vi "Compare_One_Term_Heirarchy.vi"   [LabVIEW 2021]
uses:
  Support/Equal 0/DBL/Equal 0_DBL.lvclass
  Support/Equal 0/SGL/Equal 0_SGL.lvclass
  Support/Equal 0/EXT/Equal 0_EXT.lvclass
  Support/Equal 0/CPLX_SGL/Equal 0_CPLX_SGL.lvclass
  Support/Equal 0/CPLX_DBL/Equal 0_CPLX_DBL.lvclass
  Support/Equal 0/CPLX_EXT/Equal 0_CPLX_EXT.lvclass
  Support/Equal 0/I8/Equal 0_I8.lvclass
  Support/Equal 0/I16/Equal 0_I16.lvclass
  Support/Equal 0/I32/Equal 0_I32.lvclass
  Support/Equal 0/I64/Equal 0_I64.lvclass
  Support/Equal 0/U8/Equal 0_U8.lvclass
  Support/Equal 0/U16/Equal 0_U16.lvclass
  Support/Equal 0/U32/Equal 0_U32.lvclass
  Support/Equal 0/U64/Equal 0_U64.lvclass
  Support/Less 0/DBL/Less 0_DBL.lvclass
  Support/Not Equal 0/DBL/Not Equal 0_DBL.lvclass
  Support/Greater 0/DBL/Greater 0_DBL.lvclass
  Support/Greater Equal 0/DBL/Greater Equal 0_DBL.lvclass
  Support/Lesser Equal 0/DBL/Lesser Equal 0_DBL.lvclass
  Support/Not Equal 0/SGL/Not Equal 0_SGL.lvclass
  Support/Not Equal 0/EXT/Not Equal 0_EXT.lvclass
  Support/Not Equal 0/CPLX_SGL/Not Equal 0_CPLX_SGL.lvclass
  Support/Not Equal 0/CPLX_DBL/Not Equal 0_CPLX_DBL.lvclass
  Support/Not Equal 0/CPLX_EXT/Not Equal 0_CPLX_EXT.lvclass
  Support/Not Equal 0/I8/Not Equal 0_I8.lvclass
  Support/Not Equal 0/I16/Not Equal 0_I16.lvclass
  Support/Not Equal 0/I32/Not Equal 0_I32.lvclass
  Support/Not Equal 0/I64/Not Equal 0_I64.lvclass
  Support/Not Equal 0/U8/Not Equal 0_U8.lvclass
  Support/Not Equal 0/U16/Not Equal 0_U16.lvclass
  Support/Not Equal 0/U32/Not Equal 0_U32.lvclass
  Support/Not Equal 0/U64/Not Equal 0_U64.lvclass
  Support/Greater 0/SGL/Greater 0_SGL.lvclass
  Support/Greater 0/EXT/Greater 0_EXT.lvclass
  Support/Greater 0/I8/Greater 0_I8.lvclass
  Support/Greater 0/I16/Greater 0_I16.lvclass
  Support/Greater 0/I32/Greater 0_I32.lvclass
  Support/Greater 0/I64/Greater 0_I64.lvclass
  Support/Greater 0/U8/Greater 0_U8.lvclass
  Support/Greater 0/U16/Greater 0_U16.lvclass
  Support/Greater 0/U32/Greater 0_U32.lvclass
  Support/Greater 0/U64/Greater 0_U64.lvclass
  Support/Less 0/SGL/Less 0_SGL.lvclass
  Support/Less 0/EXT/Less 0_EXT.lvclass
  Support/Less 0/I8/Less 0_I8.lvclass
  Support/Less 0/I16/Less 0_I16.lvclass
  Support/Less 0/I32/Less 0_I32.lvclass
  Support/Less 0/I64/Less 0_I64.lvclass
  Support/Less 0/U8/Less 0_U8.lvclass
  Support/Less 0/U16/Less 0_U16.lvclass
  Support/Less 0/U32/Less 0_U32.lvclass
  Support/Less 0/U64/Less 0_U64.lvclass
  Support/Greater Equal 0/SGL/Greater Equal 0_SGL.lvclass
  Support/Greater Equal 0/EXT/Greater Equal 0_EXT.lvclass
  Support/Greater Equal 0/I8/Greater Equal 0_I8.lvclass
  Support/Greater Equal 0/I16/Greater Equal 0_I16.lvclass
  Support/Greater Equal 0/I32/Greater Equal 0_I32.lvclass
  Support/Greater Equal 0/I64/Greater Equal 0_I64.lvclass
  Support/Greater Equal 0/U8/Greater Equal 0_U8.lvclass
  Support/Greater Equal 0/U16/Greater Equal 0_U16.lvclass
  Support/Greater Equal 0/U32/Greater Equal 0_U32.lvclass
  Support/Greater Equal 0/U64/Greater Equal 0_U64.lvclass
  Support/Lesser Equal 0/SGL/Lesser Equal 0_SGL.lvclass
  Support/Lesser Equal 0/EXT/Lesser Equal 0_EXT.lvclass
  Support/Lesser Equal 0/I8/Lesser Equal 0_I8.lvclass
  Support/Lesser Equal 0/I16/Lesser Equal 0_I16.lvclass
  Support/Lesser Equal 0/I32/Lesser Equal 0_I32.lvclass
  Support/Lesser Equal 0/I64/Lesser Equal 0_I64.lvclass
  Support/Lesser Equal 0/U8/Lesser Equal 0_U8.lvclass
  Support/Lesser Equal 0/U16/Lesser Equal 0_U16.lvclass
  Support/Lesser Equal 0/U32/Lesser Equal 0_U32.lvclass
  Support/Lesser Equal 0/U64/Lesser Equal 0_U64.lvclass
  Support/Compare/One Term/SGL/AbsComp_One Term_SGL.lvclass
  Support/Compare/One Term/CPLX_SGL/AbsComp_One Term_CPLX_SGL.lvclass
  Support/Compare/One Term/DBL/AbsComp_One Term_DBL.lvclass
  Support/Compare/One Term/EXT/AbsComp_One Term_EXT.lvclass
  Support/Compare/One Term/CPLX_DBL/AbsComp_One Term_CPLX_DBL.lvclass
  Support/Compare/One Term/CPLX_EXT/AbsComp_One Term_CPLX_EXT.lvclass
  Support/Compare/One Term/I8/AbsComp_One Term_I8.lvclass
  Support/Compare/One Term/I16/AbsComp_One Term_I16.lvclass
  Support/Compare/One Term/I32/AbsComp_One Term_I32.lvclass
  Support/Compare/One Term/I64/AbsComp_One Term_I64.lvclass
  Support/Compare/One Term/U8/AbsComp_One Term_U8.lvclass
  Support/Compare/One Term/U16/AbsComp_One Term_U16.lvclass
  Support/Compare/One Term/U32/AbsComp_One Term_U32.lvclass
  Support/Compare/One Term/U64/AbsComp_One Term_U64.lvclass
panel:
  # "SEE DIAGRAM\nFOR Hierarchy"
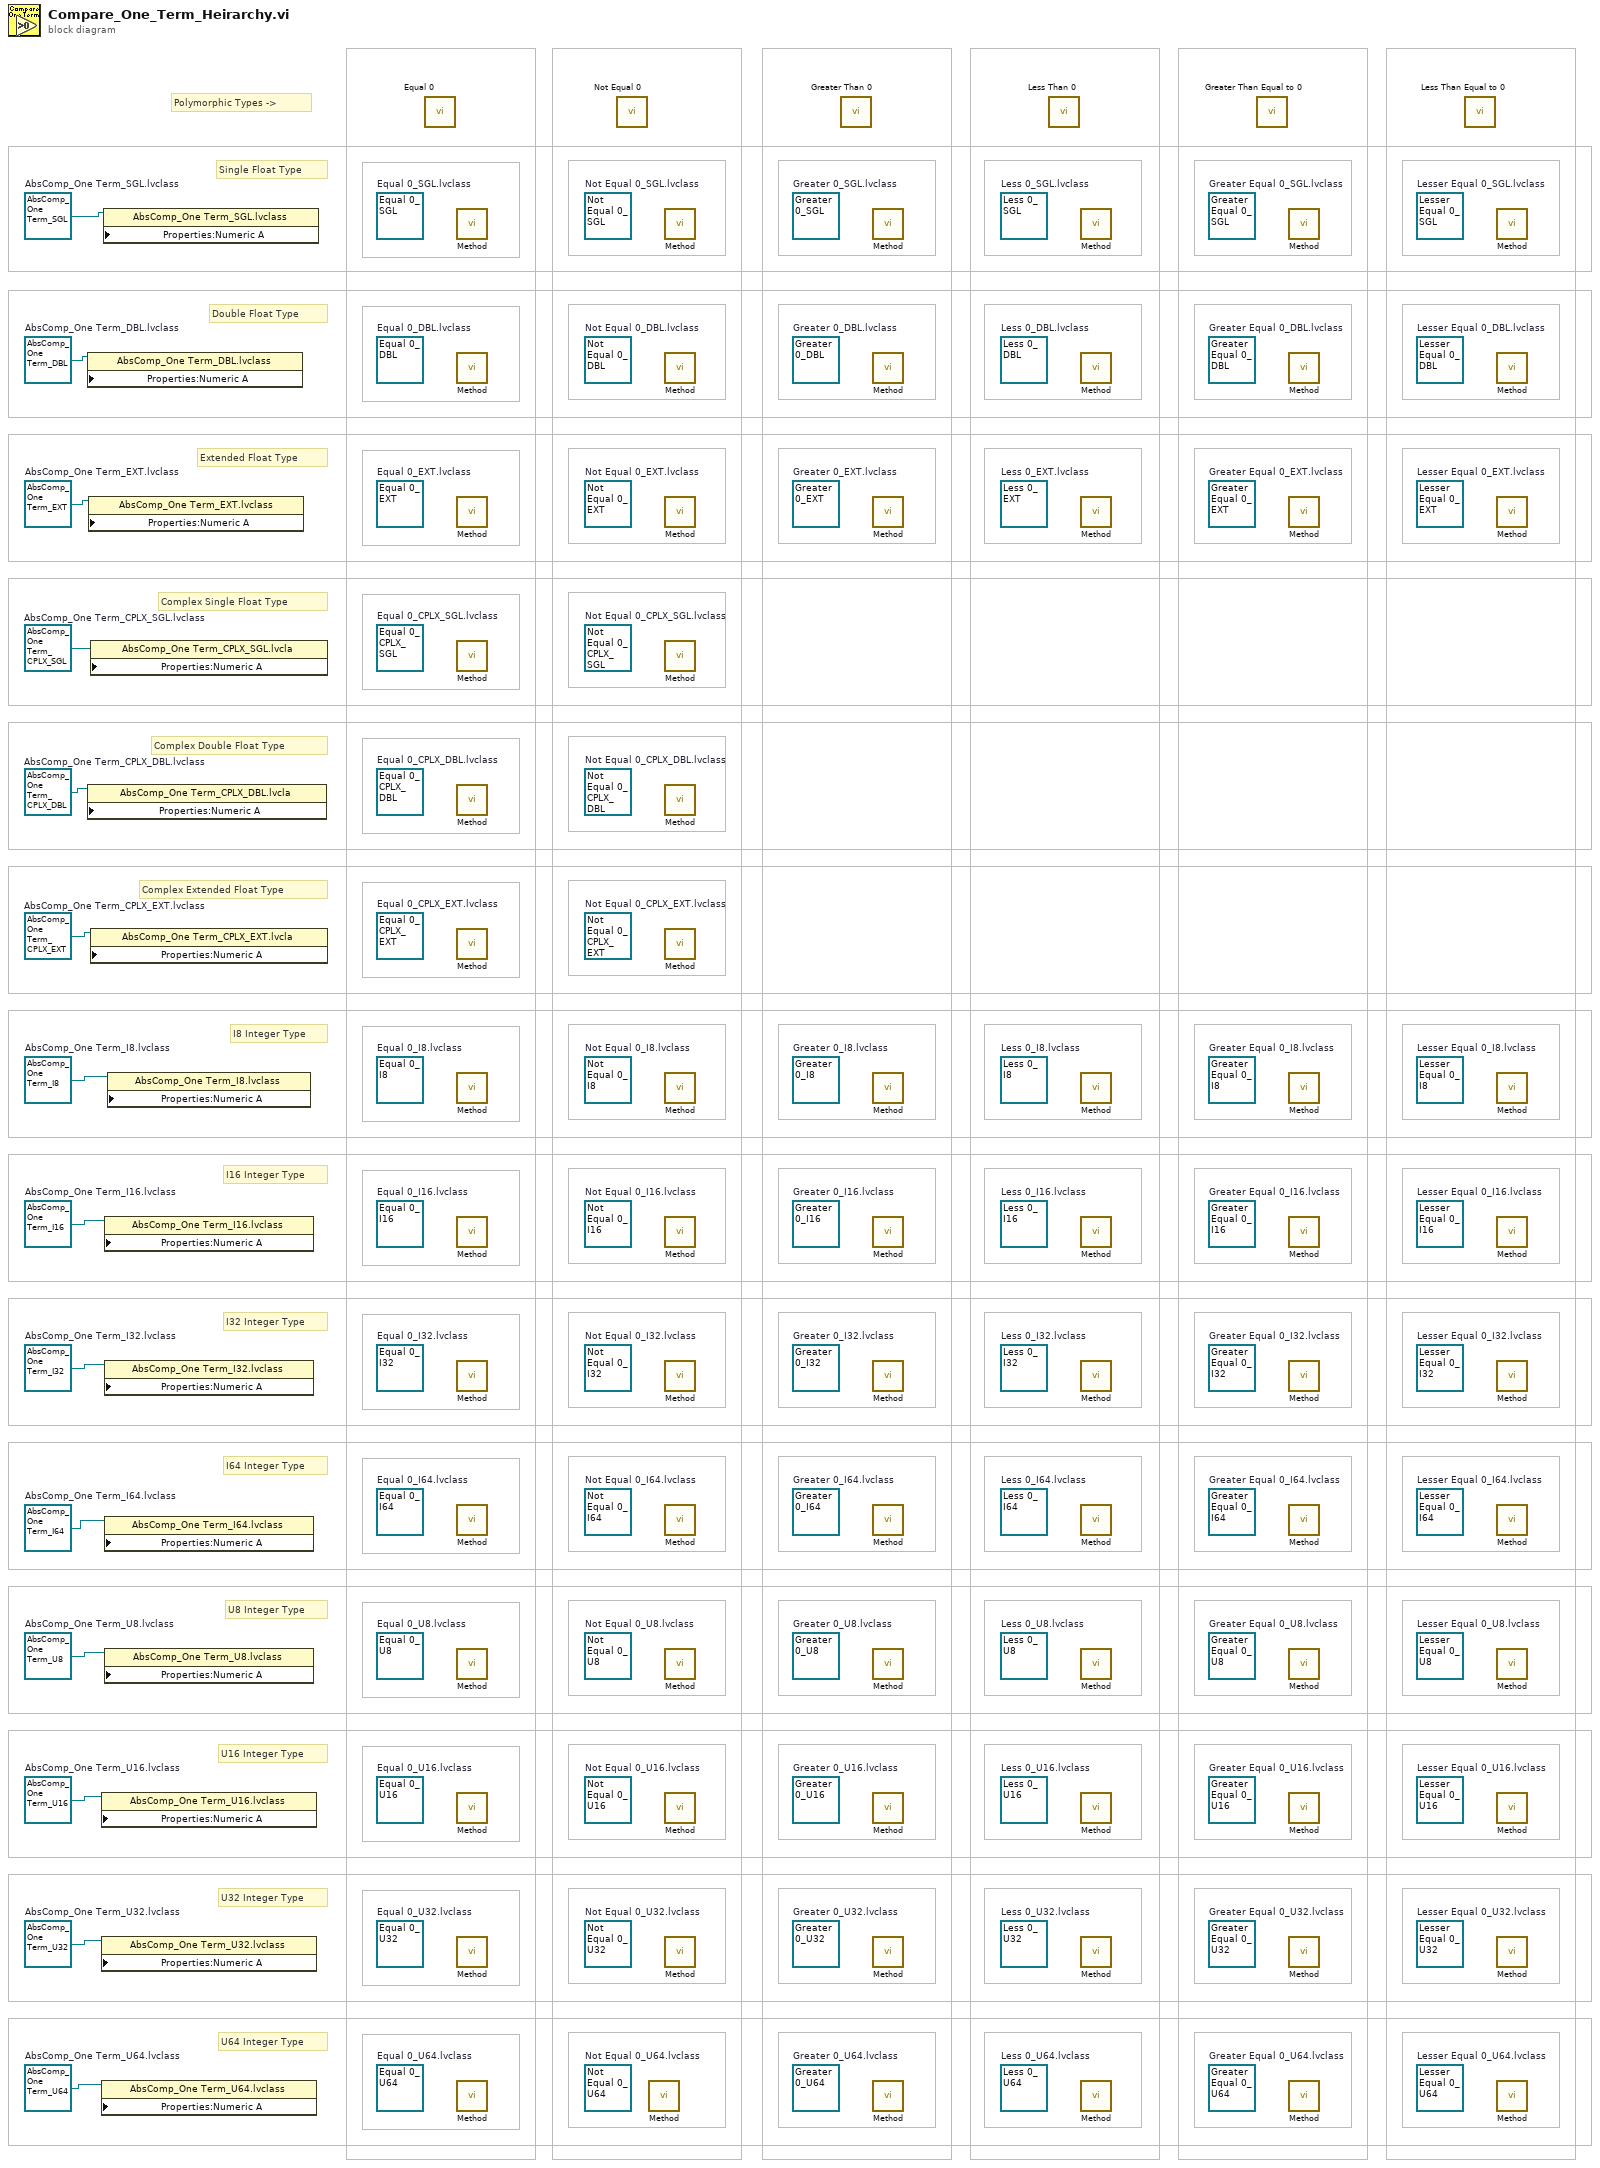
[diagram p0: block diagram]
diagram:
  w9 = refnum<class "AbsComp_One Term_U64.lvclass"> refnum  # AbsComp_One Term_U64.lvclass
  w8 = refnum<class "AbsComp_One Term_U32.lvclass"> refnum  # AbsComp_One Term_U32.lvclass
  w7 = refnum<class "AbsComp_One Term_U16.lvclass"> refnum  # AbsComp_One Term_U16.lvclass
  w6 = refnum<class "AbsComp_One Term_U8.lvclass"> refnum  # AbsComp_One Term_U8.lvclass
  w5 = refnum<class "AbsComp_One Term_I64.lvclass"> refnum  # AbsComp_One Term_I64.lvclass
  w4 = refnum<class "AbsComp_One Term_I32.lvclass"> refnum  # AbsComp_One Term_I32.lvclass
  w3 = refnum<class "AbsComp_One Term_I16.lvclass"> refnum  # AbsComp_One Term_I16.lvclass
  w2 = refnum<class "AbsComp_One Term_I8.lvclass"> refnum  # AbsComp_One Term_I8.lvclass
  w1 = refnum<class "AbsComp_One Term_CPLX_EXT.lvclass"> refnum  # AbsComp_One Term_CPLX_EXT.lvclass
  w10 = refnum<class "AbsComp_One Term_CPLX_DBL.lvclass"> refnum  # AbsComp_One Term_CPLX_DBL.lvclass
  w11 = refnum<class "AbsComp_One Term_EXT.lvclass"> refnum  # AbsComp_One Term_EXT.lvclass
  w12 = refnum<class "AbsComp_One Term_DBL.lvclass"> refnum  # AbsComp_One Term_DBL.lvclass
  w13 = refnum<class "AbsComp_One Term_CPLX_SGL.lvclass"> refnum  # AbsComp_One Term_CPLX_SGL.lvclass
  w14 = refnum<class "AbsComp_One Term_SGL.lvclass"> refnum  # AbsComp_One Term_SGL.lvclass
  (unwired) refnum<class "Lesser Equal 0_U64.lvclass"> refnum  # Lesser Equal 0_U64.lvclass
  (unwired) refnum<class "Lesser Equal 0_U32.lvclass"> refnum  # Lesser Equal 0_U32.lvclass
  (unwired) refnum<class "Lesser Equal 0_U16.lvclass"> refnum  # Lesser Equal 0_U16.lvclass
  (unwired) refnum<class "Lesser Equal 0_U8.lvclass"> refnum  # Lesser Equal 0_U8.lvclass
  (unwired) refnum<class "Lesser Equal 0_I64.lvclass"> refnum  # Lesser Equal 0_I64.lvclass
  (unwired) refnum<class "Lesser Equal 0_I32.lvclass"> refnum  # Lesser Equal 0_I32.lvclass
  (unwired) refnum<class "Lesser Equal 0_I16.lvclass"> refnum  # Lesser Equal 0_I16.lvclass
  (unwired) refnum<class "Lesser Equal 0_I8.lvclass"> refnum  # Lesser Equal 0_I8.lvclass
  (unwired) refnum<class "Lesser Equal 0_EXT.lvclass"> refnum  # Lesser Equal 0_EXT.lvclass
  (unwired) refnum<class "Lesser Equal 0_SGL.lvclass"> refnum  # Lesser Equal 0_SGL.lvclass
  (unwired) refnum<class "Lesser Equal 0_DBL.lvclass"> refnum  # Lesser Equal 0_DBL.lvclass
  (unwired) refnum<class "Greater Equal 0_U64.lvclass"> refnum  # Greater Equal 0_U64.lvclass
  (unwired) refnum<class "Greater Equal 0_U32.lvclass"> refnum  # Greater Equal 0_U32.lvclass
  (unwired) refnum<class "Greater Equal 0_U16.lvclass"> refnum  # Greater Equal 0_U16.lvclass
  (unwired) refnum<class "Greater Equal 0_U8.lvclass"> refnum  # Greater Equal 0_U8.lvclass
  (unwired) refnum<class "Greater Equal 0_I64.lvclass"> refnum  # Greater Equal 0_I64.lvclass
  (unwired) refnum<class "Greater Equal 0_I32.lvclass"> refnum  # Greater Equal 0_I32.lvclass
  (unwired) refnum<class "Greater Equal 0_I16.lvclass"> refnum  # Greater Equal 0_I16.lvclass
  (unwired) refnum<class "Greater Equal 0_I8.lvclass"> refnum  # Greater Equal 0_I8.lvclass
  (unwired) refnum<class "Greater Equal 0_EXT.lvclass"> refnum  # Greater Equal 0_EXT.lvclass
  (unwired) refnum<class "Greater Equal 0_DBL.lvclass"> refnum  # Greater Equal 0_DBL.lvclass
  (unwired) refnum<class "Greater Equal 0_SGL.lvclass"> refnum  # Greater Equal 0_SGL.lvclass
  (unwired) refnum<class "Less 0_U64.lvclass"> refnum  # Less 0_U64.lvclass
  (unwired) refnum<class "Less 0_U32.lvclass"> refnum  # Less 0_U32.lvclass
  (unwired) refnum<class "Less 0_U16.lvclass"> refnum  # Less 0_U16.lvclass
  (unwired) refnum<class "Less 0_U8.lvclass"> refnum  # Less 0_U8.lvclass
  (unwired) refnum<class "Less 0_I64.lvclass"> refnum  # Less 0_I64.lvclass
  (unwired) refnum<class "Less 0_I32.lvclass"> refnum  # Less 0_I32.lvclass
  (unwired) refnum<class "Less 0_I16.lvclass"> refnum  # Less 0_I16.lvclass
  (unwired) refnum<class "Less 0_I8.lvclass"> refnum  # Less 0_I8.lvclass
  (unwired) refnum<class "Less 0_EXT.lvclass"> refnum  # Less 0_EXT.lvclass
  (unwired) refnum<class "Less 0_DBL.lvclass"> refnum  # Less 0_DBL.lvclass
  (unwired) refnum<class "Less 0_SGL.lvclass"> refnum  # Less 0_SGL.lvclass
  (unwired) refnum<class "Greater 0_U64.lvclass"> refnum  # Greater 0_U64.lvclass
  (unwired) refnum<class "Greater 0_U32.lvclass"> refnum  # Greater 0_U32.lvclass
  (unwired) refnum<class "Greater 0_U16.lvclass"> refnum  # Greater 0_U16.lvclass
  (unwired) refnum<class "Greater 0_U8.lvclass"> refnum  # Greater 0_U8.lvclass
  (unwired) refnum<class "Greater 0_I64.lvclass"> refnum  # Greater 0_I64.lvclass
  (unwired) refnum<class "Greater 0_I32.lvclass"> refnum  # Greater 0_I32.lvclass
  (unwired) refnum<class "Greater 0_I16.lvclass"> refnum  # Greater 0_I16.lvclass
  (unwired) refnum<class "Greater 0_I8.lvclass"> refnum  # Greater 0_I8.lvclass
  (unwired) refnum<class "Greater 0_EXT.lvclass"> refnum  # Greater 0_EXT.lvclass
  (unwired) refnum<class "Greater 0_DBL.lvclass"> refnum  # Greater 0_DBL.lvclass
  (unwired) refnum<class "Greater 0_SGL.lvclass"> refnum  # Greater 0_SGL.lvclass
  (unwired) refnum<class "Not Equal 0_U64.lvclass"> refnum  # Not Equal 0_U64.lvclass
  (unwired) refnum<class "Not Equal 0_U32.lvclass"> refnum  # Not Equal 0_U32.lvclass
  (unwired) refnum<class "Not Equal 0_U16.lvclass"> refnum  # Not Equal 0_U16.lvclass
  (unwired) refnum<class "Not Equal 0_U8.lvclass"> refnum  # Not Equal 0_U8.lvclass
  (unwired) refnum<class "Not Equal 0_I64.lvclass"> refnum  # Not Equal 0_I64.lvclass
  (unwired) refnum<class "Not Equal 0_I32.lvclass"> refnum  # Not Equal 0_I32.lvclass
  (unwired) refnum<class "Not Equal 0_I16.lvclass"> refnum  # Not Equal 0_I16.lvclass
  (unwired) refnum<class "Not Equal 0_I8.lvclass"> refnum  # Not Equal 0_I8.lvclass
  (unwired) refnum<class "Not Equal 0_CPLX_EXT.lvclass"> refnum  # Not Equal 0_CPLX_EXT.lvclass
  (unwired) refnum<class "Not Equal 0_CPLX_DBL.lvclass"> refnum  # Not Equal 0_CPLX_DBL.lvclass
  (unwired) refnum<class "Not Equal 0_CPLX_SGL.lvclass"> refnum  # Not Equal 0_CPLX_SGL.lvclass
  (unwired) refnum<class "Not Equal 0_EXT.lvclass"> refnum  # Not Equal 0_EXT.lvclass
  (unwired) refnum<class "Not Equal 0_DBL.lvclass"> refnum  # Not Equal 0_DBL.lvclass
  (unwired) refnum<class "Not Equal 0_SGL.lvclass"> refnum  # Not Equal 0_SGL.lvclass
  (unwired) refnum<class "Equal 0_U64.lvclass"> refnum  # Equal 0_U64.lvclass
  (unwired) refnum<class "Equal 0_U32.lvclass"> refnum  # Equal 0_U32.lvclass
  (unwired) refnum<class "Equal 0_U16.lvclass"> refnum  # Equal 0_U16.lvclass
  (unwired) refnum<class "Equal 0_U8.lvclass"> refnum  # Equal 0_U8.lvclass
  (unwired) refnum<class "Equal 0_I64.lvclass"> refnum  # Equal 0_I64.lvclass
  (unwired) refnum<class "Equal 0_I32.lvclass"> refnum  # Equal 0_I32.lvclass
  (unwired) refnum<class "Equal 0_I16.lvclass"> refnum  # Equal 0_I16.lvclass
  (unwired) refnum<class "Equal 0_I8.lvclass"> refnum  # Equal 0_I8.lvclass
  (unwired) refnum<class "Equal 0_CPLX_EXT.lvclass"> refnum  # Equal 0_CPLX_EXT.lvclass
  (unwired) refnum<class "Equal 0_CPLX_DBL.lvclass"> refnum  # Equal 0_CPLX_DBL.lvclass
  (unwired) refnum<class "Equal 0_CPLX_SGL.lvclass"> refnum  # Equal 0_CPLX_SGL.lvclass
  (unwired) refnum<class "Equal 0_EXT.lvclass"> refnum  # Equal 0_EXT.lvclass
  (unwired) refnum<class "Equal 0_DBL.lvclass"> refnum  # Equal 0_DBL.lvclass
  (unwired) refnum<class "Equal 0_SGL.lvclass"> refnum  # Equal 0_SGL.lvclass
  # "Polymorphic Types ->"
  # "U64 Integer Type"
  # "U32 Integer Type"
  # "U16 Integer Type"
  # "U8 Integer Type"
  # "I64 Integer Type"
  # "I32 Integer Type"
  # "I16 Integer Type"
  # "I8 Integer Type"
  # "Complex Extended Float Type"
  # "Complex Double Float Type"
  # "Complex Single Float Type"
  # "Extended Float Type"
  # "Double Float Type"
  # "Single Float Type"
  n1 = property class="AbsComp_One Term_DBL.lvclass" props=["Properties:Numeric A"](reference=w12) -> ()  [unwired: 2 in, 2 out]
  n2 = property class="AbsComp_One Term_CPLX_DBL.lvcla" props=["Properties:Numeric A"](reference=w10) -> ()  [unwired: 2 in, 2 out]
  n3 = property class="AbsComp_One Term_EXT.lvclass" props=["Properties:Numeric A"](reference=w11) -> ()  [unwired: 2 in, 2 out]
  n4 = property class="AbsComp_One Term_CPLX_SGL.lvcla" props=["Properties:Numeric A"](reference=w13) -> ()  [unwired: 2 in, 2 out]
  n5 = property class="AbsComp_One Term_CPLX_EXT.lvcla" props=["Properties:Numeric A"](reference=w1) -> ()  [unwired: 2 in, 2 out]
  n6 = property class="AbsComp_One Term_U16.lvclass" props=["Properties:Numeric A"](reference=w7) -> ()  [unwired: 2 in, 2 out]
  n7 = property class="AbsComp_One Term_U32.lvclass" props=["Properties:Numeric A"](reference=w8) -> ()  [unwired: 2 in, 2 out]
  n8 = property class="AbsComp_One Term_U64.lvclass" props=["Properties:Numeric A"](reference=w9) -> ()  [unwired: 2 in, 2 out]
  n9 = property class="AbsComp_One Term_SGL.lvclass" props=["Properties:Numeric A"](reference=w14) -> ()  [unwired: 2 in, 2 out]
  n10 = property class="AbsComp_One Term_I16.lvclass" props=["Properties:Numeric A"](reference=w3) -> ()  [unwired: 2 in, 2 out]
  n11 = property class="AbsComp_One Term_I32.lvclass" props=["Properties:Numeric A"](reference=w4) -> ()  [unwired: 2 in, 2 out]
  n12 = property class="AbsComp_One Term_I64.lvclass" props=["Properties:Numeric A"](reference=w5) -> ()  [unwired: 2 in, 2 out]
  n13 = property class="AbsComp_One Term_U8.lvclass" props=["Properties:Numeric A"](reference=w6) -> ()  [unwired: 2 in, 2 out]
  n14 = property class="AbsComp_One Term_I8.lvclass" props=["Properties:Numeric A"](reference=w2) -> ()  [unwired: 2 in, 2 out]
  n15 = call-poly "Equal 0.vi"() -> ()  [unwired: 5 in, 1 out]
  n16 = call "Method.vi"() -> ()  [unwired: 5 in, 1 out]
  n17 = call "Method.vi"() -> ()  [unwired: 5 in, 1 out]
  n18 = call "Method.vi"() -> ()  [unwired: 5 in, 1 out]
  n19 = call "Method.vi"() -> ()  [unwired: 5 in, 1 out]
  n20 = call "Method.vi"() -> ()  [unwired: 5 in, 1 out]
  n21 = call "Method.vi"() -> ()  [unwired: 5 in, 1 out]
  n22 = call "Method.vi"() -> ()  [unwired: 5 in, 1 out]
  n23 = call "Method.vi"() -> ()  [unwired: 5 in, 1 out]
  n24 = call "Method.vi"() -> ()  [unwired: 5 in, 1 out]
  n25 = call "Method.vi"() -> ()  [unwired: 5 in, 1 out]
  n26 = call "Method.vi"() -> ()  [unwired: 5 in, 1 out]
  n27 = call "Method.vi"() -> ()  [unwired: 5 in, 1 out]
  n28 = call "Method.vi"() -> ()  [unwired: 5 in, 1 out]
  n29 = call "Method.vi"() -> ()  [unwired: 5 in, 1 out]
  n30 = call-poly "Not Equal 0.vi"() -> ()  [unwired: 5 in, 1 out]
  n31 = call "Method.vi"() -> ()  [unwired: 5 in, 1 out]
  n32 = call "Method.vi"() -> ()  [unwired: 5 in, 1 out]
  n33 = call "Method.vi"() -> ()  [unwired: 5 in, 1 out]
  n34 = call "Method.vi"() -> ()  [unwired: 5 in, 1 out]
  n35 = call "Method.vi"() -> ()  [unwired: 5 in, 1 out]
  n36 = call "Method.vi"() -> ()  [unwired: 5 in, 1 out]
  n37 = call "Method.vi"() -> ()  [unwired: 5 in, 1 out]
  n38 = call "Method.vi"() -> ()  [unwired: 5 in, 1 out]
  n39 = call "Method.vi"() -> ()  [unwired: 5 in, 1 out]
  n40 = call "Method.vi"() -> ()  [unwired: 5 in, 1 out]
  n41 = call "Method.vi"() -> ()  [unwired: 5 in, 1 out]
  n42 = call "Method.vi"() -> ()  [unwired: 5 in, 1 out]
  n43 = call "Method.vi"() -> ()  [unwired: 5 in, 1 out]
  n44 = call "Method.vi"() -> ()  [unwired: 5 in, 1 out]
  n45 = call-poly "Greater Than 0.vi"() -> ()  [unwired: 5 in, 1 out]
  n46 = call "Method.vi"() -> ()  [unwired: 5 in, 1 out]
  n47 = call "Method.vi"() -> ()  [unwired: 5 in, 1 out]
  n48 = call "Method.vi"() -> ()  [unwired: 5 in, 1 out]
  n49 = call "Method.vi"() -> ()  [unwired: 5 in, 1 out]
  n50 = call "Method.vi"() -> ()  [unwired: 5 in, 1 out]
  n51 = call "Method.vi"() -> ()  [unwired: 5 in, 1 out]
  n52 = call "Method.vi"() -> ()  [unwired: 5 in, 1 out]
  n53 = call "Method.vi"() -> ()  [unwired: 5 in, 1 out]
  n54 = call "Method.vi"() -> ()  [unwired: 5 in, 1 out]
  n55 = call "Method.vi"() -> ()  [unwired: 5 in, 1 out]
  n56 = call "Method.vi"() -> ()  [unwired: 5 in, 1 out]
  n57 = call-poly "Less Than 0.vi"() -> ()  [unwired: 5 in, 1 out]
  n58 = call "Method.vi"() -> ()  [unwired: 5 in, 1 out]
  n59 = call "Method.vi"() -> ()  [unwired: 5 in, 1 out]
  n60 = call "Method.vi"() -> ()  [unwired: 5 in, 1 out]
  n61 = call "Method.vi"() -> ()  [unwired: 5 in, 1 out]
  n62 = call "Method.vi"() -> ()  [unwired: 5 in, 1 out]
  n63 = call "Method.vi"() -> ()  [unwired: 5 in, 1 out]
  n64 = call "Method.vi"() -> ()  [unwired: 5 in, 1 out]
  n65 = call "Method.vi"() -> ()  [unwired: 5 in, 1 out]
  n66 = call "Method.vi"() -> ()  [unwired: 5 in, 1 out]
  n67 = call "Method.vi"() -> ()  [unwired: 5 in, 1 out]
  n68 = call "Method.vi"() -> ()  [unwired: 5 in, 1 out]
  n69 = call-poly "Greater Than Equal to 0.vi"() -> ()  [unwired: 5 in, 1 out]
  n70 = call "Method.vi"() -> ()  [unwired: 5 in, 1 out]
  n71 = call "Method.vi"() -> ()  [unwired: 5 in, 1 out]
  n72 = call "Method.vi"() -> ()  [unwired: 5 in, 1 out]
  n73 = call "Method.vi"() -> ()  [unwired: 5 in, 1 out]
  n74 = call "Method.vi"() -> ()  [unwired: 5 in, 1 out]
  n75 = call "Method.vi"() -> ()  [unwired: 5 in, 1 out]
  n76 = call "Method.vi"() -> ()  [unwired: 5 in, 1 out]
  n77 = call "Method.vi"() -> ()  [unwired: 5 in, 1 out]
  n78 = call "Method.vi"() -> ()  [unwired: 5 in, 1 out]
  n79 = call "Method.vi"() -> ()  [unwired: 5 in, 1 out]
  n80 = call "Method.vi"() -> ()  [unwired: 5 in, 1 out]
  n81 = call-poly "Less Than Equal to 0.vi"() -> ()  [unwired: 5 in, 1 out]
  n82 = call "Method.vi"() -> ()  [unwired: 5 in, 1 out]
  n83 = call "Method.vi"() -> ()  [unwired: 5 in, 1 out]
  n84 = call "Method.vi"() -> ()  [unwired: 5 in, 1 out]
  n85 = call "Method.vi"() -> ()  [unwired: 5 in, 1 out]
  n86 = call "Method.vi"() -> ()  [unwired: 5 in, 1 out]
  n87 = call "Method.vi"() -> ()  [unwired: 5 in, 1 out]
  n88 = call "Method.vi"() -> ()  [unwired: 5 in, 1 out]
  n89 = call "Method.vi"() -> ()  [unwired: 5 in, 1 out]
  n90 = call "Method.vi"() -> ()  [unwired: 5 in, 1 out]
  n91 = call "Method.vi"() -> ()  [unwired: 5 in, 1 out]
  n92 = call "Method.vi"() -> ()  [unwired: 5 in, 1 out]
